vi "Module - Login.vi"(8 "Error In":errorcluster) -> (0 "Error Out":errorcluster)   [LabVIEW 2020]
uses:
  Control/State - Module Login.ctl
  Control/State - eFGV.ctl
  Control/State - FGV.ctl
  Control/Header - User Management.ctl
  Control/Header - Page.ctl
panel:
  in  "Cancel":bool
  in  "Password:":string
  in  "Username:":string
  in  "Login":bool
  in  "Stop":bool
  # "Please login to continue . . ."
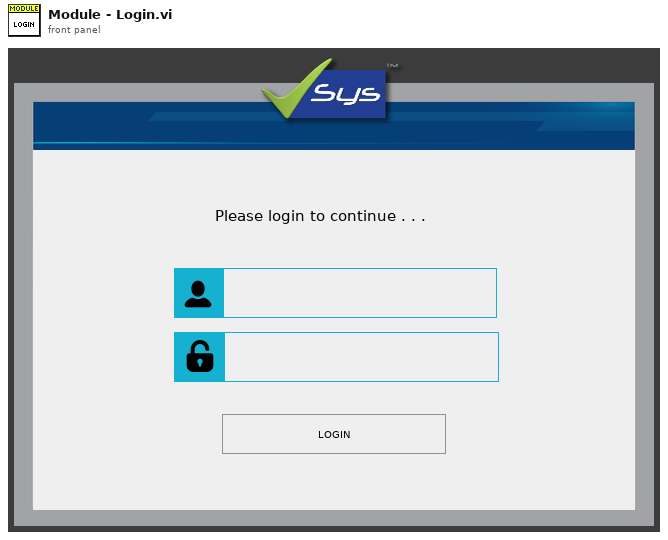
[diagram p1: front panel]
types:
  T1 = cluster{"T_Out":i32, "Login?":bool, "Username":string, "Selected User Index":i32}
  T2 = typedef "State - Module Login.ctl" = enum16{"Init", "Register Event", "Idle", "Login", "Update Page", "Close"}
  T3 = typedef "State - eFGV.ctl" = enum16{"Init", "Read", "Write", "Exit"}
  T4 = typedef "Header - User Management.ctl" = enum16{"Name", "Staff ID", "Username", "Password", "Access Level", "Status", "Access Page"}
  T5 = typedef "State - FGV.ctl" = enum16{"Write", "Read"}
  T6 = typedef "Header - Page.ctl" = enum16{"P1 Main", "P2", "P3 Analysis", "P4 Prediction", "P5 User"}
  T7 = typedef "License File Parameter.ctl" = cluster{"Expired Time":string, "Computer ID":string, "Product Name":string, "Period":i16, "Activated Time":string, "License Level":enum16{"Level 1", "Level 2", "Level 3", "Level 4", "Level 5"}, "License Type":enum16{"Free", "Trial", "Subscription", "Perpetual"}, "Log Time":string}
  T8 = enum16{"Level 1", "Level 2", "Level 3", "Level 4", "Level 5"}
  T9 = typedef "Page List Configuration.ctl" = cluster{"HMI Configuration":cluster{"EXE Name":string, "Project Name":string, "Max Page No":i32, "HMI State":enum32{"Invalid", "Standard", "Closed", "Hidden", "Minimized", "Maximized"}, "Version":enum16{"Demo", "User"}, "Check License":bool, "Font Size":u32, "Res: Height":i16, "Res: Width":i16, "License Level":enum16{"Level 1", "Level 2", "Level 3", "Level 4", "Level 5"}, "License Type":enum16{"Free", "Trial", "Subscription", "Perpetual"}}, "All HMI Module":string[], "Default HMI Module":string[], "Page Module":string[], "Page List: Level 1":string[], "Page List: Level 2":string[], "Page List: Level 3":string[], "All RT Module":string[], "Default RT Module":string[], "Acquire Enable Page":string[], "Log Enable Page":string[], "Run Page":string[], "Kill Page":string[], "Button":cluster{"Text":string[], "Tip Strip":string[]}}
  T10 = enum32{"invalid app kind", "Development System", "Run Time System", "Student Edition", "Embedded LabVIEW", "Evaluation", "Custom"}
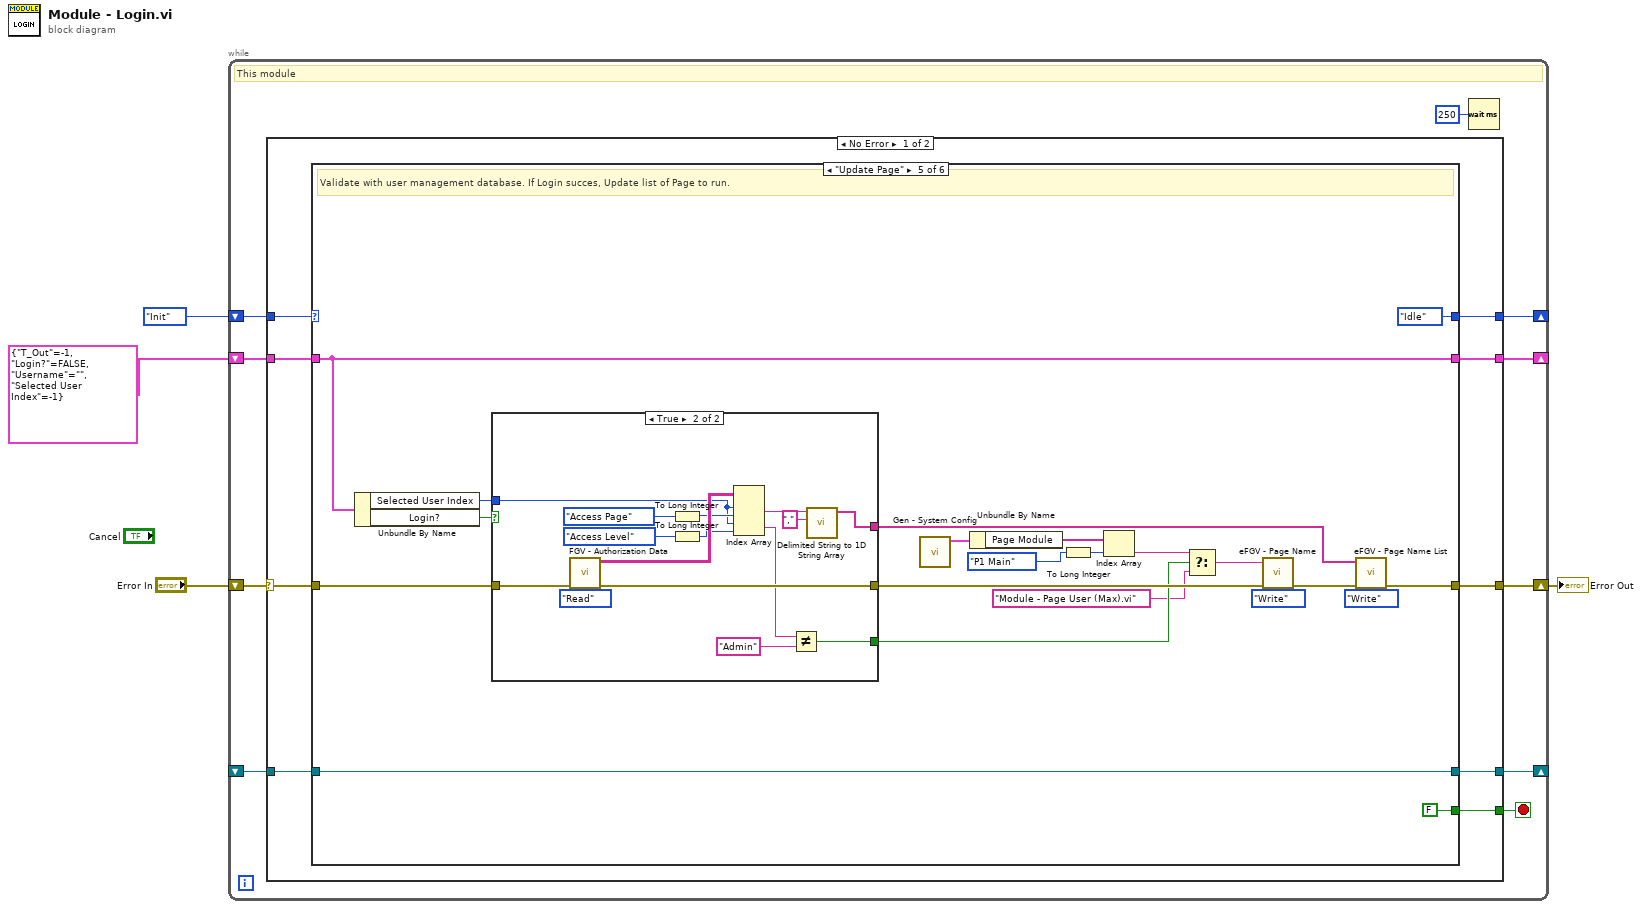
[diagram p0: block diagram]
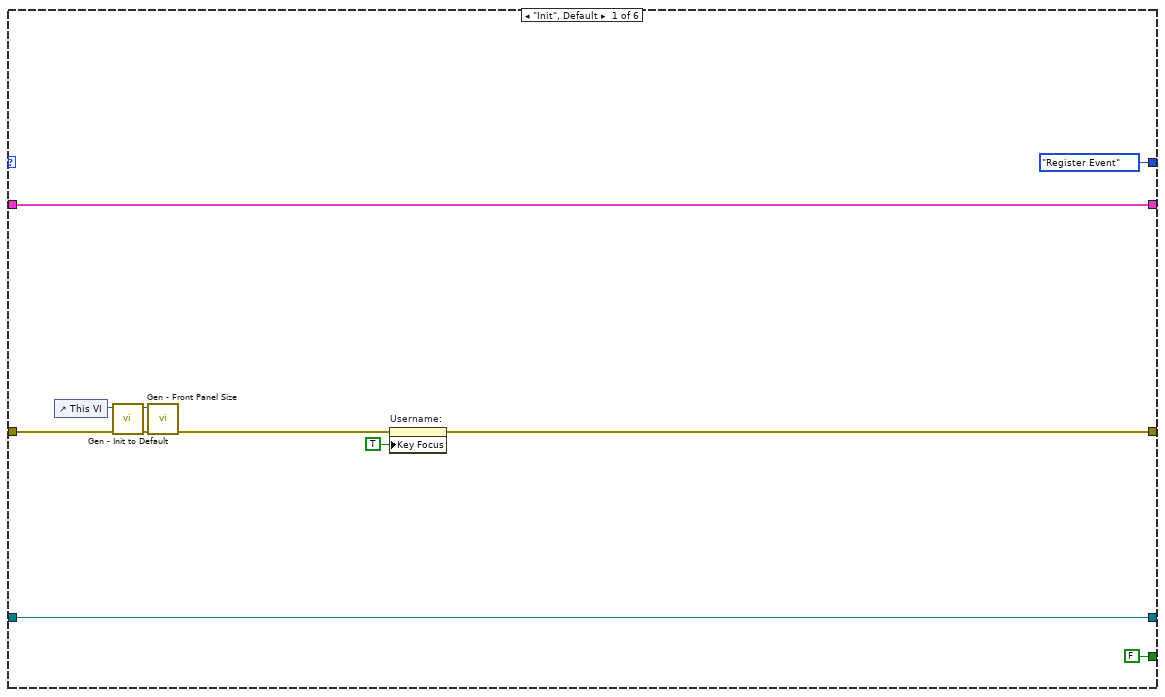
[diagram p2: hidden frame]
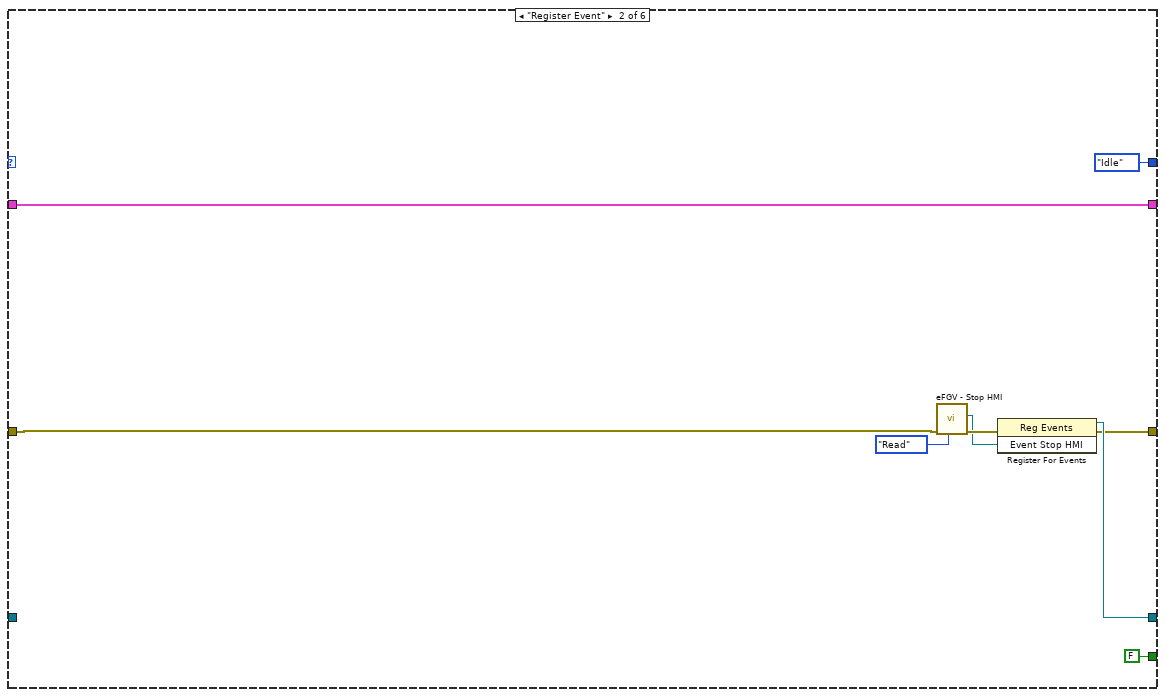
[diagram p3: hidden frame]
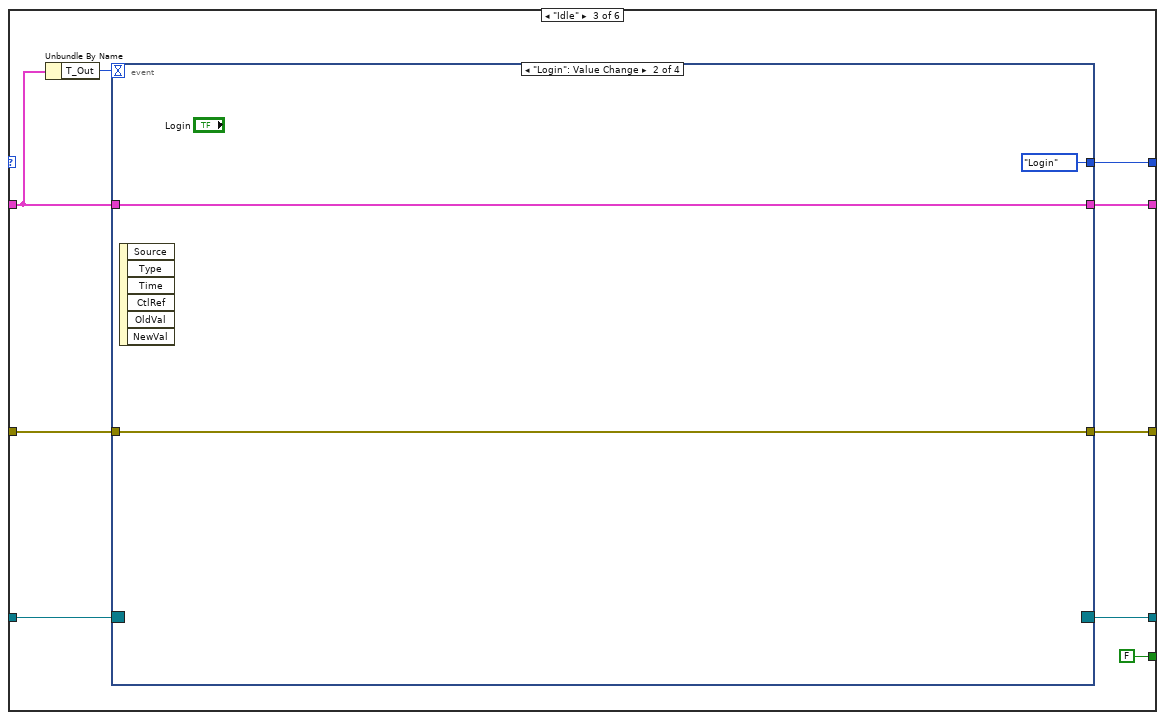
[diagram p4: hidden frame]
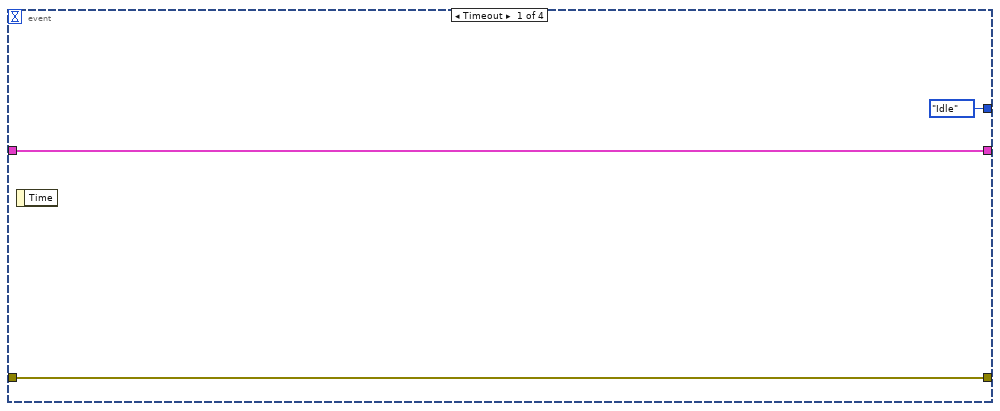
[diagram p5: hidden frame]
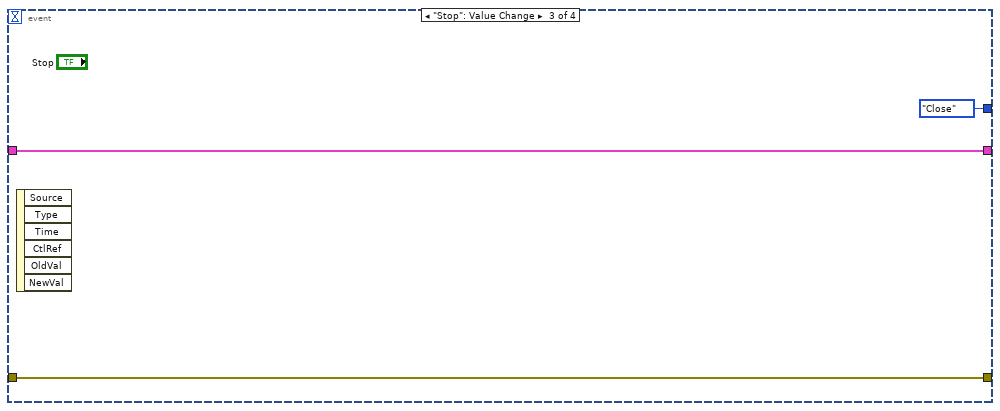
[diagram p6: hidden frame]
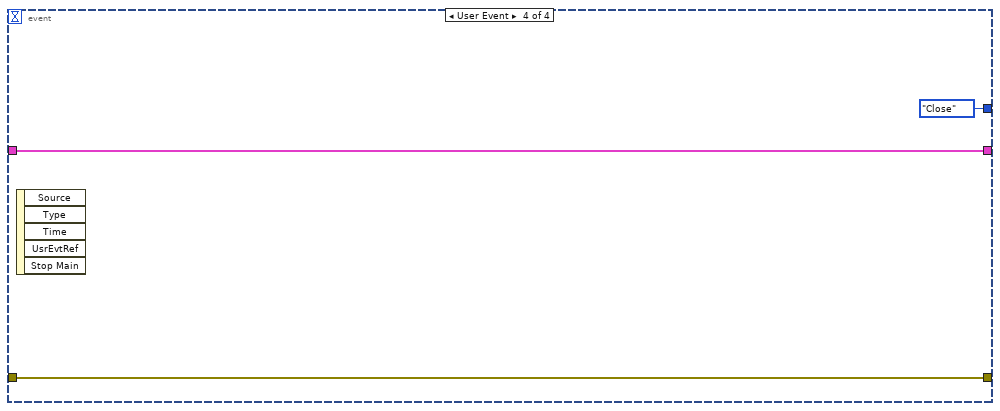
[diagram p7: hidden frame]
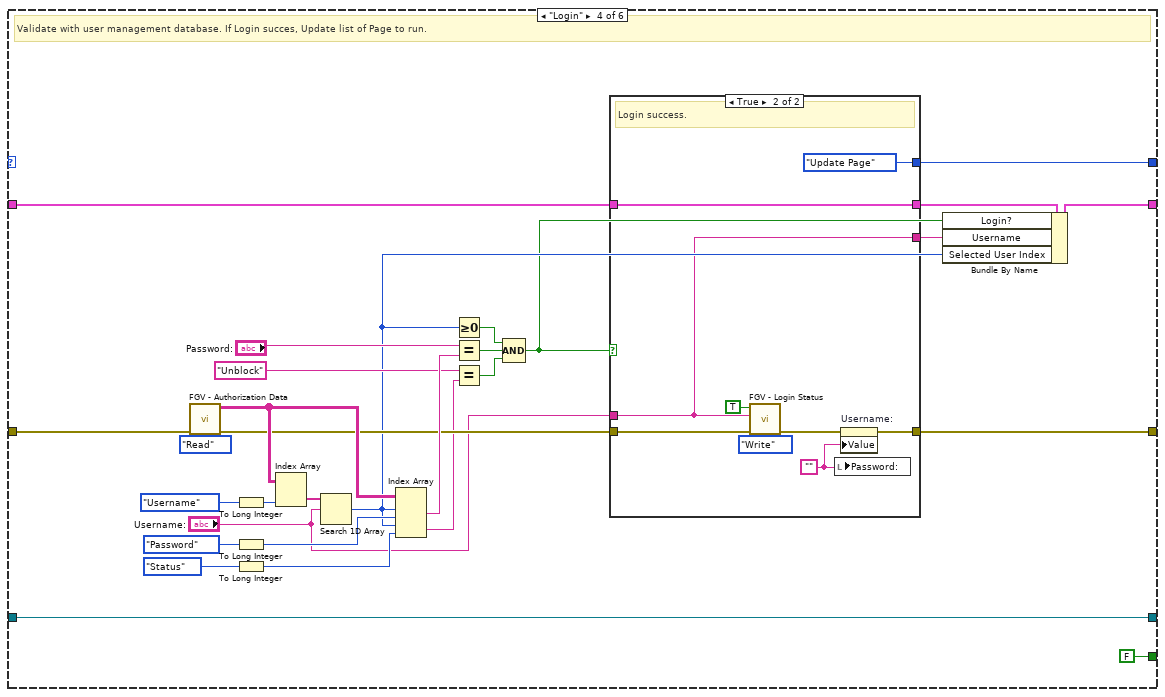
[diagram p8: hidden frame]
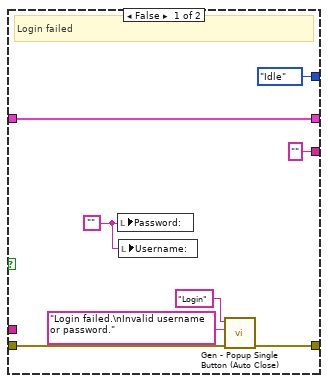
[diagram p9: hidden frame]
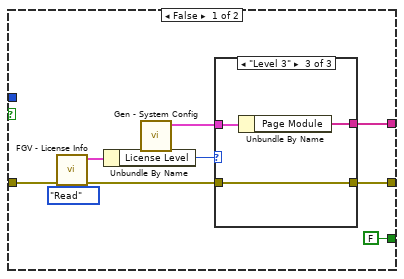
[diagram p10: hidden frame]
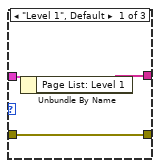
[diagram p11: hidden frame]
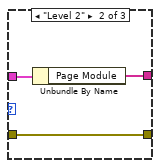
[diagram p12: hidden frame]
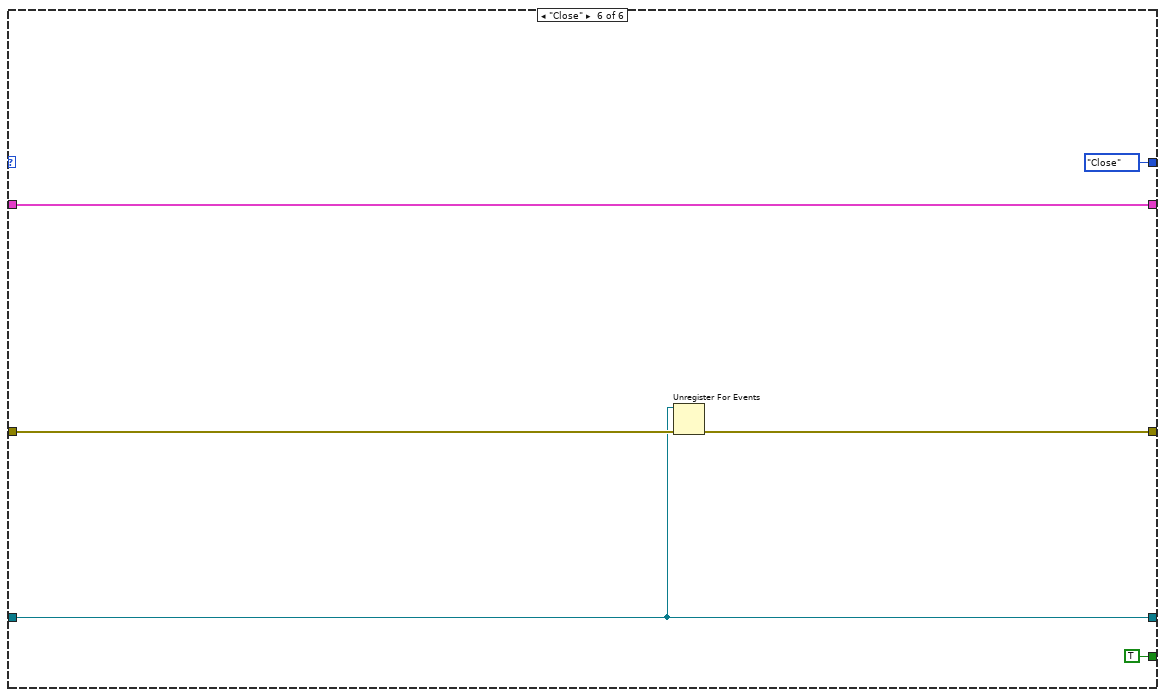
[diagram p13: hidden frame]
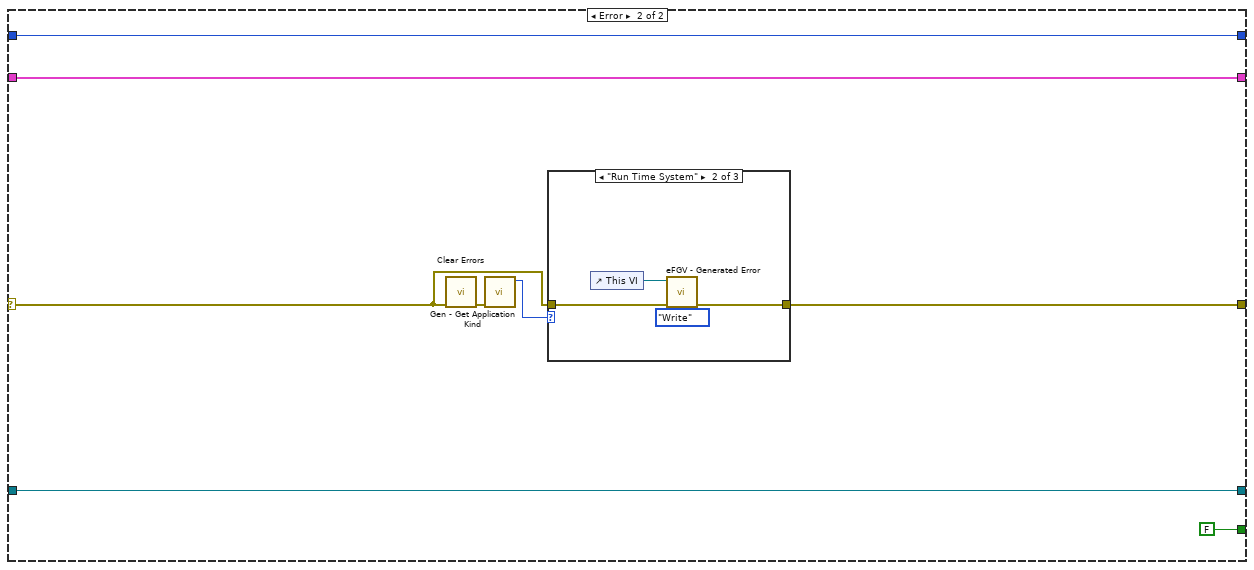
[diagram p14: hidden frame]
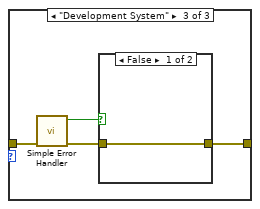
[diagram p16: hidden frame]
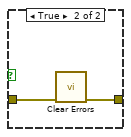
[diagram p17: hidden frame]
diagram:
  n1 = while {
    shift-right: [w5] -> _
    shift-left: State_-_Module_Login."Init" -> [w12]
    shift-right: [w13] -> w3
    shift-left: "Error In" -> [w14]
    shift-right: [w10] -> _
    shift-left: _ -> [w9]
    shift-right: [w7] -> _
    shift-left: T1 {"T_Out"=-1, "Login?"=FALSE, "Username"="", "Selected User Index"=-1} -> [w8]
    stop <- w11 stop-if-true
    # "This module"
    n2 = case shown="No Error" w14 {
      selector: w14 -> [w22 w172]
      tunnel: w12 -> [w21 w175]
      tunnel: [w23 w171] -> w13
      tunnel: [w20 FALSE] -> w11
      tunnel: [w19 w177] -> w10
      tunnel: w9 -> [w18 w177]
      tunnel: w8 -> [w17 w176]
      tunnel: [w16 w176] -> w7
      tunnel: [w15 w175] -> w5
      frame No Error {
        n3 = case shown="\"Update Page\"" w21 {
          tunnel: [w27 w38 w52 w90 w121 w169] -> w23
          tunnel: w22 -> [w34 w43 w51 w88 w126 w170]
          tunnel: [FALSE FALSE FALSE FALSE FALSE TRUE] -> w20
          tunnel: [w30 w40 w48 w92 w130 w167] -> w19
          tunnel: w18 -> [w30 _ w49 w92 w130 w167]
          tunnel: w17 -> [w32 w42 w46 w69 w125 w168]
          tunnel: [w32 w42 w47 w68 w125 w168] -> w16
          tunnel: [State_-_Module_Login."Register Event" State_-_Module_Login."Idle" w44 w83 State_-_Module_Login."Idle" State_-_Module_Login."Close"] -> w15
          frame "Init", Default {
            n4 = control-ref of="This VI"() -> (w24:refnum<vi>)
            n5 = call "Gen - Init to Default.vi"("Error in"=w34, "This VI"=w24) -> ("Error out"=w33:errorcluster, "This VI Copy"=w25:refnum<vi>)  [unwired: 8 in]
            n6 = call "Gen - Front Panel Size.vi"("Error In"=w33, "This VI"=w25) -> ("Error Out"=w28:errorcluster)  [unwired: 9 in]
            n7 = property on="Username:" class="Str"(error in=w28, "Key Focus"=TRUE) -> (error out=w27:errorcluster)  [unwired: 1 in, 1 out]
          }
          frame "Register Event" {
            n8 = call "eFGV - Stop HMI.vi"("Action"=State_-_eFGV."Read", "Error In"=w43) -> ("Error Out"=w39:errorcluster, "Event Stop HMI"=w36:refnum<user-event>)  [unwired: 7 in, 1 out]
            n9 = register-events(error in=w39, w36) -> (reference out=w40:refnum<event-registration>, error out=w38:errorcluster)  [unwired: 1 in]
          }
          frame "Idle" {
            n10 = Unbundle By Name(w46) -> ("T_Out"=w45:i32)
            n11 = event shown="[1] \"Login\": Value Change" {
              selector: w49 -> [_ _ _ _]
              dyn-events: [_ _ _ _] -> w48
              timeout: w45 -> [_ _ _ _]
              tunnel: [w55 w58 w61 w64] -> w52
              tunnel: w51 -> [w55 w58 w61 w64]
              tunnel: [w54 w57 w60 w63] -> w47
              tunnel: w46 -> [w54 w57 w60 w63]
              tunnel: [State_-_Module_Login."Idle" State_-_Module_Login."Login" State_-_Module_Login."Close" State_-_Module_Login."Close"] -> w44
              event Timeout {
                n12 = event-data() -> ()  [unwired: 1 in, 1 out]
              }
              event "Login": Value Change {
                n13 = event-data() -> ()  [unwired: 1 in, 6 out]
              }
              event "Stop": Value Change {
                n14 = event-data() -> ()  [unwired: 1 in, 6 out]
              }
              event User Event {
                n15 = event-data() -> ()  [unwired: 1 in, 5 out]
              }
            }
          }
          frame "Login" {
            # "Validate with user management database. If Login succes, Update list of Page to run."
            n16 = call "FGV - Authorization Data.vi"("State - FGV"=State_-_FGV."Read", "Error In"=w88) -> ("Error Out"=w84:errorcluster, "Data Out"=w86:string[][])  [unwired: 8 in]
            n17 = To Long Integer(number=Header_-_User_Management."Username" ("Header - User Management")) -> (32bit integer=w80:i32)
            n18 = To Long Integer(number=Header_-_User_Management."Password" ("Header - User Management")) -> (32bit integer=w79:i32)
            n19 = To Long Integer(number=Header_-_User_Management."Status" ("Header - User Management")) -> (32bit integer=w77:i32)
            n20 = Index Array(array=w86, index (col)=w80) -> (element=w87:string[])  [unwired: 1 in]
            n21 = Search 1D Array(1D array=w87, element="Username:") -> (index of element=w66:i32)  [unwired: 1 in]
            n22 = Index Array(array=w86, index (row) #1=w66, index (col) #1=w79, index (row) #2=w66, index (col) #2=w77) -> (element #1=w85:string, element #2=w74:string)
            n23 = Greater Or Equal To 0?(x=w66) -> (x >= 0?=w76:bool)
            n24 = Equal?(x="Password:", y=w85) -> (x = y?=w75:bool)
            n25 = Equal?(x="Unblock", y=w74) -> (x = y?=w72:bool)
            n26 = Compound Arithmetic op=AND(w76, w75, w72) -> (w65:bool)
            n27 = case shown="True" w65 {
              tunnel: [w100 w105] -> w90
              tunnel: w84 -> [w101 w108]
              tunnel: [State_-_Module_Login."Idle" State_-_Module_Login."Update Page"] -> w83
              tunnel: "Username:" -> [_ w102]
              tunnel: [w95 w107] -> w70
              tunnel: w69 -> [w95 w107]
              tunnel: ["" ("Username:") w102] -> w67
              frame False {
                w96 = ""
                # "Login failed"
                n28 = local write "Password:"(w96) -> ()
                n29 = local write "Username:"(w96) -> ()
                n30 = call "Gen - Popup Single Button (Auto Close).vi"("Error in"=w101, "Message in"="Login failed.\nInvalid username or password.", "Header"="Login") -> ("Error out"=w100:errorcluster)  [unwired: 7 in, 1 out]
              }
              frame True {
                w104 = ""
                # "Login success."
                n31 = call "FGV - Login Status.vi"("Action"=enum16{"Read", "Write"}."Write", "Error In"=w108, "Username in"=w102, "Login In"=TRUE) -> ("Error Out"=w103:errorcluster)  [unwired: 5 in, 2 out]
                n32 = local write "Password:"(w104) -> ()
                n33 = property on="Username:" class="Str"(error in=w103, "Value"=w104) -> (error out=w105:errorcluster)  [unwired: 1 in, 1 out]
              }
            }
            n34 = Bundle By Name(cluster=w70, "Login?"=w65, "Username"=w67, "Selected User Index"=w66) -> (w68:T1)
          }
          frame "Update Page" {
            # "Validate with user management database. If Login succes, Update list of Page to run."
            n35 = Unbundle By Name(w125) -> ("Selected User Index"=w123:i32, "Login?"=w124:bool)
            n36 = case shown="True" w124 {
              tunnel: w126 -> [w136 w164]
              tunnel: [w134 w157] -> w119
              tunnel: [w133 w163] -> w128
              tunnel: w123 -> [_ w155]
              tunnel: [FALSE w150] -> w114
              frame False {
                n37 = call "FGV - License Info.vi"("FGV States"=enum16{"Read", "Write"}."Read", "Error In"=w136) -> ("Error Out"=w140:errorcluster, "License Info"=w138:T7)  [unwired: 8 in]
                n38 = Unbundle By Name(w138) -> ("License Level"=w139:T8)
                n39 = call "Gen - System Config.vi"() -> ("Data Out"=w135:T9)  [unwired: 11 in]
                n40 = case shown="\"Level 3\"" w139 {
                  tunnel: [w143 w146 w149] -> w133
                  tunnel: w140 -> [w143 w146 w149]
                  tunnel: w135 -> [w142 w145 w148]
                  tunnel: [w141 w144 w147] -> w134
                  frame "Level 1", Default {
                    n41 = Unbundle By Name(w142) -> ("Page List: Level 1"=w141:string[])
                  }
                  frame "Level 2" {
                    n42 = Unbundle By Name(w145) -> ("Page Module"=w144:string[])
                  }
                  frame "Level 3" {
                    n43 = Unbundle By Name(w148) -> ("Page Module"=w147:string[])
                  }
                }
              }
              frame True {
                n44 = call "FGV - Authorization Data.vi"("State - FGV"=State_-_FGV."Read", "Error In"=w164) -> ("Error Out"=w163:errorcluster, "Data Out"=w161:string[][])  [unwired: 8 in]
                n45 = To Long Integer(number=Header_-_User_Management."Access Page" ("Header - User Management")) -> (32bit integer=w159:i32)
                n46 = To Long Integer(number=Header_-_User_Management."Access Level" ("Header - User Management")) -> (32bit integer=w153:i32)
                n47 = Index Array(array=w161, index (row) #1=w155, index (col) #1=w159, index (row) #2=w155, index (col) #2=w153) -> (element #1=w158:string, element #2=w152:string)
                n48 = Not Equal?(x=w152, y="Admin") -> (x != y?=w150:bool)
                n49 = call <vilib>:"Delimited String to 1D String Array.vi"("delimiter"=",", "delimited string"=w158) -> ("string array"=w157:string[])  [unwired: 9 in]
              }
            }
            n50 = call "Gen - System Config.vi"() -> ("Data Out"=w118:T9)  [unwired: 11 in]
            n51 = Unbundle By Name(w118) -> ("Page Module"=w117:string[])
            n52 = To Long Integer(number=Header_-_Page."P1 Main" ("f")) -> (32bit integer=w116:i32)
            n53 = Index Array(array=w117, index=w116) -> (element=w112:string)
            n54 = Select(t=w112, s=w114, f="Module - Page User (Max).vi" ("element")) -> (s? t:f=w111:string)
            n55 = call "eFGV - Page Name.vi"("Action"=State_-_eFGV."Write", "Error In"=w128, "Page Name"=w111) -> ("Error Out"=w122:errorcluster)  [unwired: 6 in, 2 out]
            n56 = call "eFGV - Page Name List.vi"("Action"=State_-_eFGV."Write", "Error In"=w122, "Enable Page In"=w119) -> ("Error Out"=w121:errorcluster)  [unwired: 6 in, 2 out]
          }
          frame "Close" {
            n57 = Unregister For Events(event registration refnum=w167, error in=w170) -> (error out=w169:errorcluster)
          }
        }
      }
      frame Error {
        n58 = call <vilib>:"Clear Errors.vi"("error in (no error)"=w172) -> ("error out"=w174:errorcluster)  [unwired: 5 in, 1 out]
        n59 = call "Gen - Get Application Kind.vi"("Error In"=w174) -> ("Application:Kind"=w173:T10)  [unwired: 9 in, 1 out]
        n60 = case shown="\"Run Time System\"" w173 {
          tunnel: [w179 w183 w187] -> w171
          tunnel: w172 -> [w179 w182 w185]
          frame "invalid app kind", Default {
          }
          frame "Run Time System" {
            n61 = control-ref of="This VI"() -> (w180:refnum<vi>)
            n62 = call "eFGV - Generated Error.vi"("eFGV States"=State_-_eFGV."Write", "Error In"=w182, "This VI"=w180) -> ("Error Out"=w183:errorcluster)  [unwired: 7 in, 1 out]
          }
          frame "Development System" {
            n63 = call <vilib>:"Simple Error Handler.vi"("error in (no error)"=w185) -> ("error?"=w184:bool, "error out"=w186:errorcluster)  [unwired: 4 in, 3 out]
            n64 = case shown="False" w184 {
              tunnel: [w188 w190] -> w187
              tunnel: w186 -> [w188 w189]
              frame False {
              }
              frame True {
                n65 = call <vilib>:"Clear Errors.vi"("error in (no error)"=w189) -> ("error out"=w190:errorcluster)  [unwired: 5 in, 1 out]
              }
            }
          }
        }
      }
    }
    n66 = Wait (ms)(milliseconds to wait=u32 250) -> ()  [unwired: 1 out]
  }
  "Error Out" <- w3
